vi "Right Joystick Get All.vi"(8 "error in (no error)":errorcluster) -> (0 "error out":errorcluster, 1 "Buttons":bool[](array[boolean]), 2 "Axes [Cluster]":T1, 3 "Axes":dbl[](array[numeric]))   [LabVIEW 2015]
uses:
  Joystick Axes Cluster.ctl
  <vilib>/Rock Robotics/WPI/Utilities/WPI_GetSetVariantRefNum.vi
  <vilib>/Rock Robotics/Network Tables/NT Write Numeric Array.vi
  <vilib>/Rock Robotics/Network Tables/NT Write Boolean Array.vi
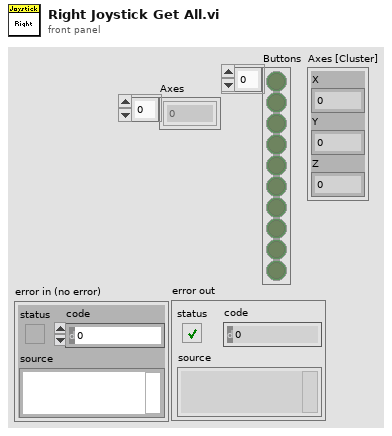
[diagram p1: front panel]
types:
  T1 = typedef "Joystick Axes Cluster.ctl" = cluster{"X":dbl, "Y":dbl, "Z":dbl}
  T2 = typedef "WPI_JoystickDevRef.ctl" = cluster{"Device":T3}
  T3 = typedef "WPI_JoystickDeviceEnum.ctl" = enum16{"USB 0", "USB 1", "USB 2", "USB 3", "USB 4", "USB 5"}
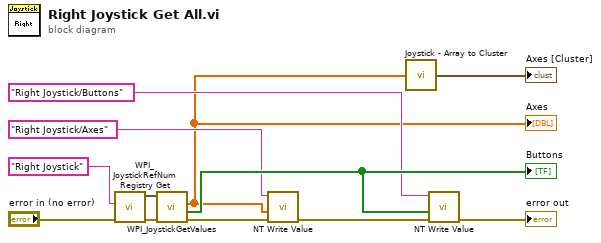
[diagram p0: block diagram]
diagram:
  n1 = call <vilib>:"WPI_JoystickRefNum Registry Get.vi"("error in (no error)"="error in (no error)", "refnum name"="Right Joystick") -> ("error out"=w7:errorcluster, "JoystickDevRef"=w8:T2)  [unwired: 8 out]
  n2 = call <vilib>:"WPI_JoystickGetValues.vi"("error in (no error)"=w7, "JoystickDevRef"=w8) -> ("error out"=w6:errorcluster, "Buttons"=w12:bool[], "Axes"=w1:dbl[])  [unwired: 5 in, 2 out]
  "Axes" <- w1
  "Buttons" <- w12
  n3 = call-poly <vilib>:"NT Write Value.vi"("error in"=w6, "Numeric Array"=w1, "Name"="Right Joystick/Axes") -> ("error out"=w5:errorcluster)  [unwired: 8 in]
  n4 = call "Joystick - Array to Cluster.vi"("Axes"=w1) -> ("Axes [Cluster]"=→"Axes [Cluster]":T1)
  n5 = call-poly <vilib>:"NT Write Value.vi"("error in"=w5, "Boolean Array"=w12, "Name"="Right Joystick/Buttons") -> ("error out"=→"error out":errorcluster)  [unwired: 8 in]
